vi "hackrf_spectrum_analyser_.vi"() -> ()   [LabVIEW 2020]
panel:
  in  "Server TCP port":dbl
  in  "Server IPv4 Address":string
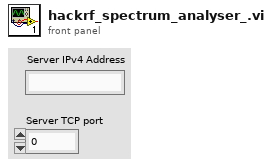
[diagram p1: front panel]
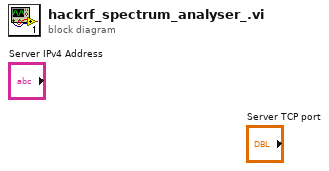
[diagram p0: block diagram]
diagram:
